vi "variant_to_binary_data.vi"(10 "error in (no error)":errorcluster, 11 "DataIn":variant) -> (2 "error out":errorcluster, 3 "binaryData":T1)   [LabVIEW 2015, in "BSON_convertors_Library.lvlib"]
uses:
  BSON_convertors_Library.lvlib
  typedefs/binaryData_cluster.ctl
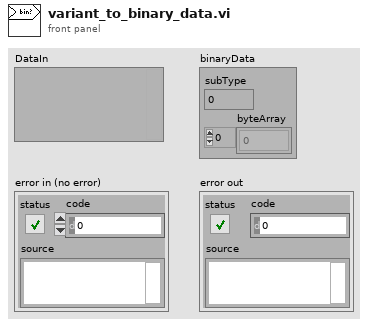
[diagram p1: front panel]
types:
  T1 = typedef "BSON_convertors_Library.lvlib/binaryData_cluster.ctl" = cluster{"subType":u8, "byteArray":u8[]}
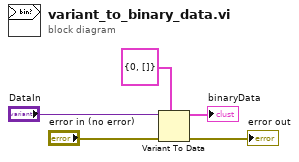
[diagram p0: block diagram]
diagram:
  n1 = Variant To Data(error in="error in (no error)", type=T1 {"subType"=0, "byteArray"=[]} ("binaryData"), Variant="DataIn") -> (data=→"binaryData":T1, error out=→"error out":errorcluster)
